vi "NewtonsPPA_Coupling.vi"(8 "error in":errorcluster, 10 "Coupling Phase 1 (AC+DC)":enum16{"AC+DC", "AC only", "DC only"}(ring), 11 "VISA.name":refnum<visa-resource-name>) -> (0 "error out":errorcluster, 3 "VISA.name out":refnum<visa-resource-name>)   [LabVIEW 2025, in "NewtonsPSM1735.lvlib"]
doc: "This VI set the coupling settings of the PPA2530"
uses:
  NewtonsPSM1735.lvlib
panel:
  in  "Coupling Pase 3 (AC+DC)":enum16{"AC+DC", "AC only", "DC only"}(ring)
  in  "Coupling Phase 2 (AC+DC)":enum16{"AC+DC", "AC only", "DC only"}(ring)
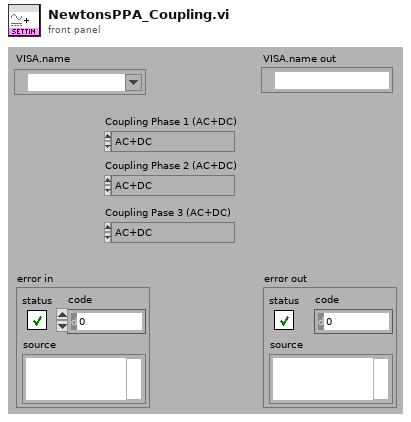
[diagram p1: front panel]
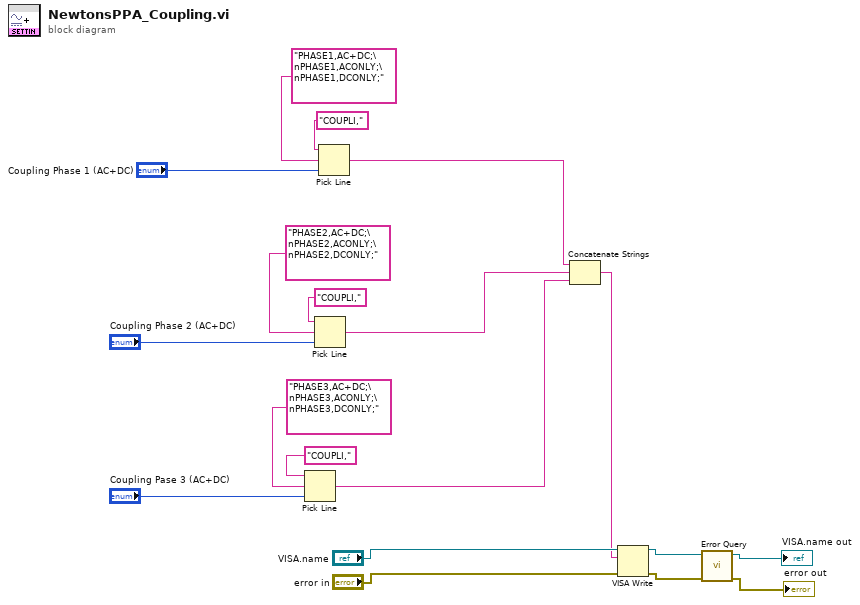
[diagram p0: block diagram]
diagram:
  n1 = Pick Line(string ("")="COUPLI,", multi-line string="PHASE3,AC+DC;\nPHASE3,ACONLY;\nPHASE3,DCONLY;", line index="Coupling Pase 3 (AC+DC)") -> (output string=w5:string)
  n2 = Pick Line(string ("")="COUPLI,", multi-line string="PHASE2,AC+DC;\nPHASE2,ACONLY;\nPHASE2,DCONLY;", line index="Coupling Phase 2 (AC+DC)") -> (output string=w6:string)
  n3 = Pick Line(string ("")="COUPLI,", multi-line string="PHASE1,AC+DC;\nPHASE1,ACONLY;\nPHASE1,DCONLY;", line index="Coupling Phase 1 (AC+DC)") -> (output string=w7:string)
  n4 = Concatenate Strings(w7, w6, w5) -> (w8:string)
  n5 = VISA Write(VISA resource name="VISA.name", write buffer=w8, error in (no error)="error in") -> (VISA resource name out=w2:refnum<visa-resource-name>, error out=w4:errorcluster)  [unwired: 1 out]
  n6 = call "Error Query.vi"("error in (no error)"=w4, "VISA resource name"=w2) -> ("error out"=→"error out":errorcluster, "VISA resource name out"=→"VISA.name out":refnum<visa-resource-name>)  [unwired: 8 out]
